vi "Logging Message Loop.vi"(8 "error in (no error)":T1 caption="entrée d'erreur (pas d'erreur)", 10 "File d'attente de données":refnum<queue>, 11 "Files d'attente de messages":T2) -> (0 "error out":T1 caption="sortie d'erreur")   [LabVIEW 2020, in "Logging.lvlib"]
doc: "Sous-VI de la boucle de messages qui gère les messages concernant l'enregistrement des données dans un fichier."
uses:
  Logging.lvlib
  support/Message Queue/All Message Queues.ctl
  support/Message Queue/Message Cluster.ctl
  Logging Configuration.ctl
  Logging State.ctl
  support/Message Queue/Enqueue Message (Single).vi
  <vilib>/Utility/error.llb/Error Cluster From Error Code.vi
  <vilib>/ErrorRing/Error Ring.xnode
  support/Message Queue/Message Queue.lvlib
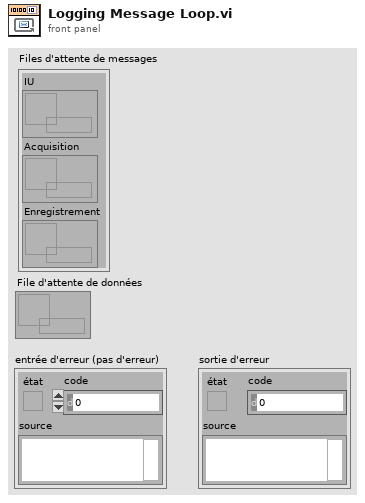
[diagram p1: front panel]
types:
  T1 = cluster{"état":bool, "code":i32, "source":string}
  T2 = typedef "Message Queue.lvlib/All Message Queues.ctl" = cluster{"IU":refnum<queue>, "Acquisition":refnum<queue>, "Enregistrement":refnum<queue>}
  T3 = typedef "Logging.lvlib/Logging Configuration.ctl" = cluster{"Chemin de base du fichier journal":path, "Référence de fichier TDMS":refnum<k34>}
  T4 = typedef "Logging.lvlib/Logging State.ctl" = enum16{"Idle", "Logging"}
  T5 = enum16{"open", "open or create", "create or replace", "create", "open (read-only)"}
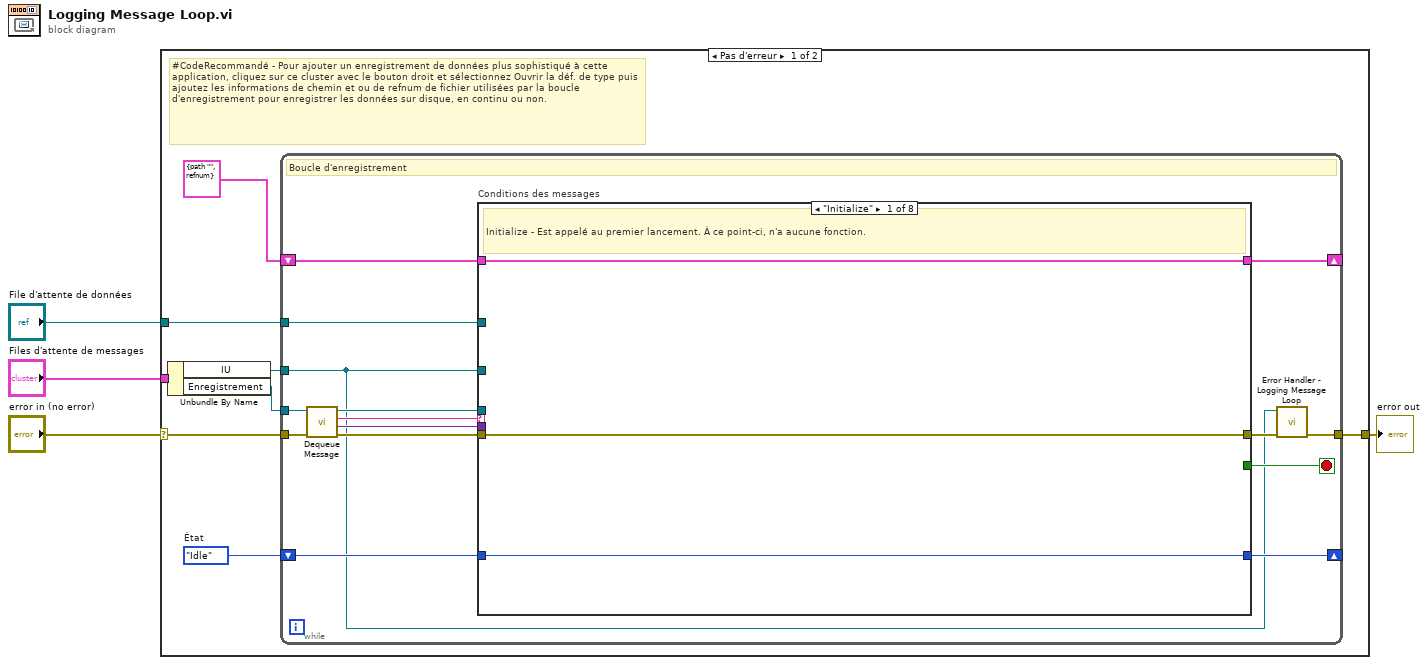
[diagram p0: block diagram]
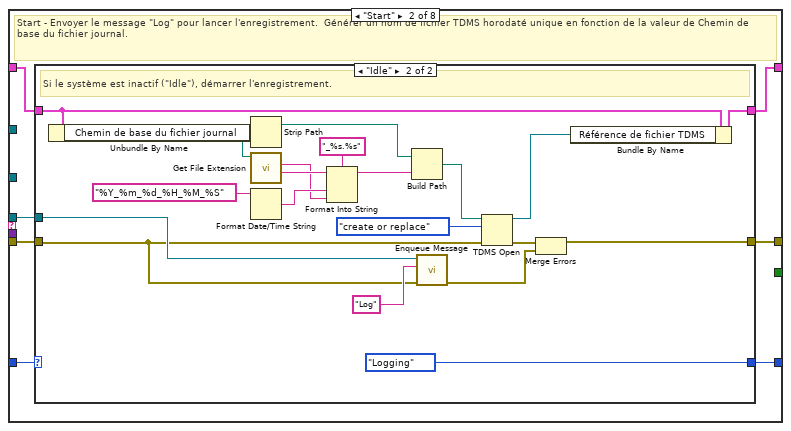
[diagram p2: hidden frame]
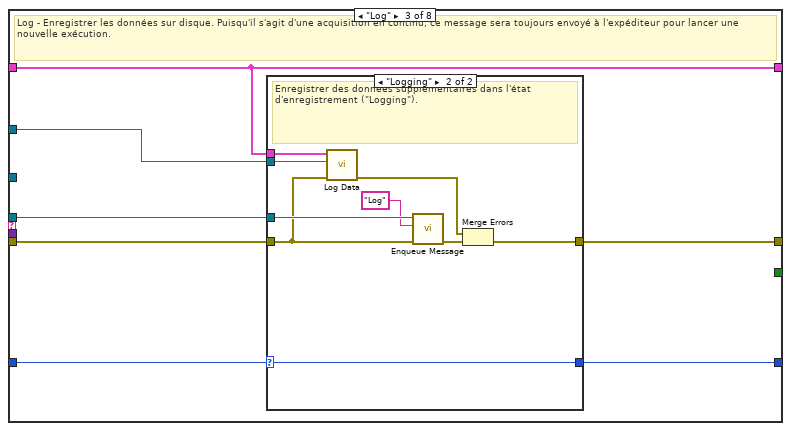
[diagram p4: hidden frame]
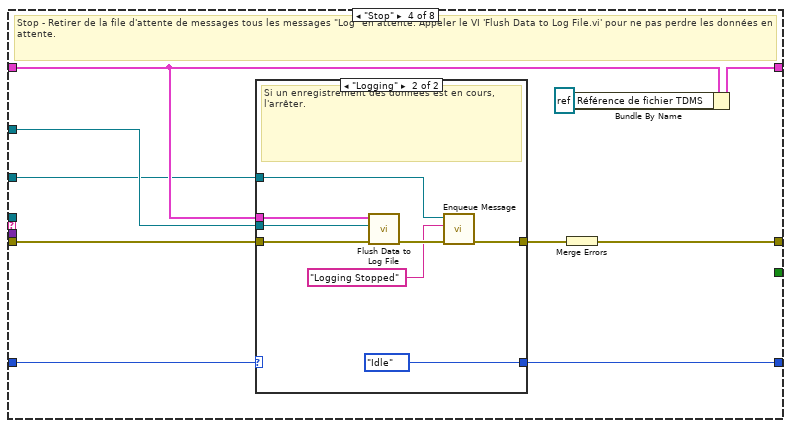
[diagram p6: hidden frame]
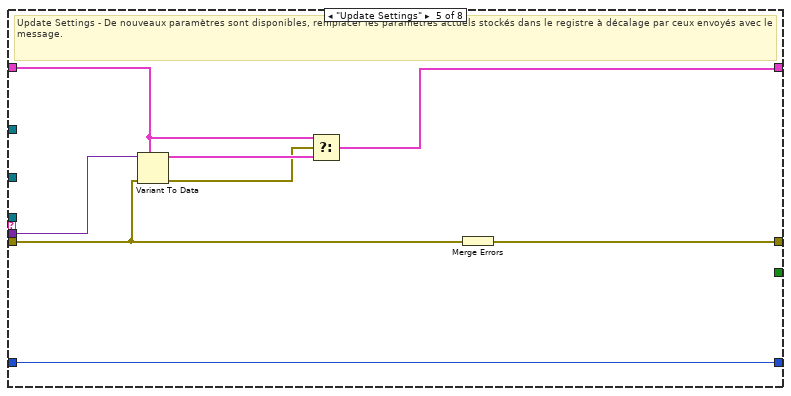
[diagram p8: hidden frame]
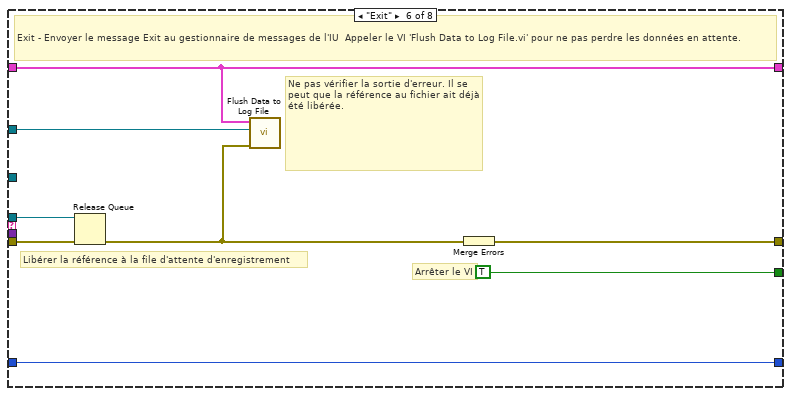
[diagram p9: hidden frame]
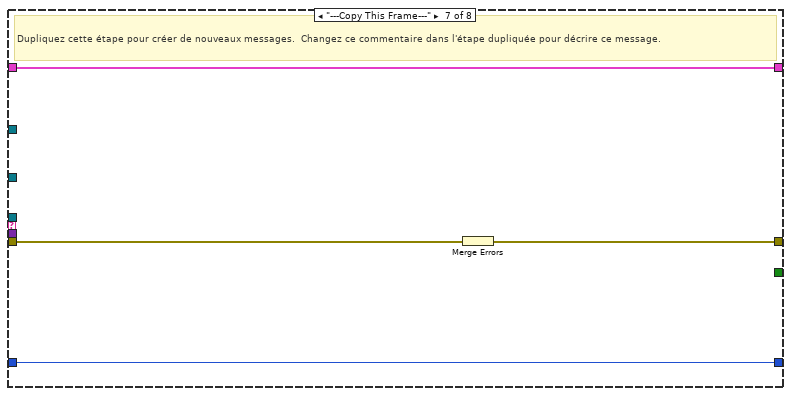
[diagram p10: hidden frame]
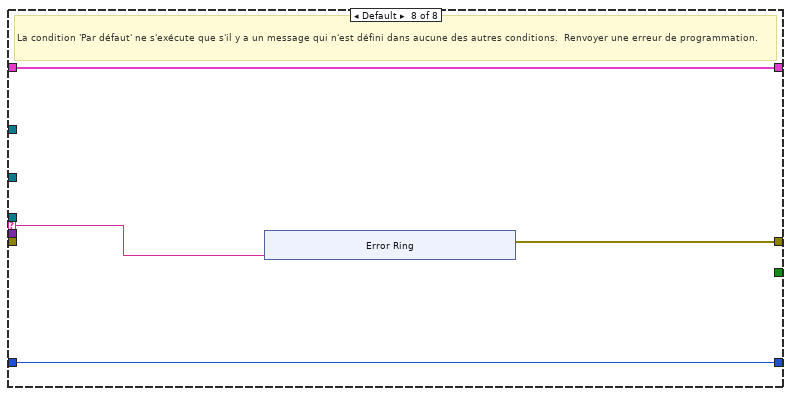
[diagram p11: hidden frame]
diagram:
  n1 = case shown="Pas d'erreur" "error in (no error)" {
    selector: "error in (no error)" -> [w8 w130]
    tunnel: "Files d'attente de messages" -> [w12 _]
    tunnel: [w10 w130] -> w3
    tunnel: "File d'attente de données" -> [w7 _]
    frame No Error {
      w5 = Logging_State."Idle"  # État
      # "#CodeRecommandé - Pour ajouter un enregistrement de données plus sophistiqué à cette application, cliquez sur ce cluster avec le bouton droit et sélectionnez Ouvrir la déf. de type puis ajoutez les informations de chemin et ou de refnum de fichier utilisées par la boucle d'enregistrement pour enregistrer les données sur disque, en continu ou non."
      n2 = Unbundle By Name(w12) -> ("IU"=w6:refnum<queue>, "Enregistrement"=w11:refnum<queue>)
      n3 = while {
        tunnel: w11 -> [w19]
        shift-right: [w26] -> _
        shift-left: T3 {"Chemin de base du fichier journal"=path "", "Référence de fichier TDMS"=refnum} ("Logging Configuration") -> [w27]
        tunnel: w6 -> [w13]
        tunnel: w7 -> [w18]
        shift-right: [w16] -> _
        shift-left: w5 -> [w17]
        tunnel: w8 -> [w24]
        tunnel: [w15] -> w10
        stop <- w25 stop-if-true
        # "Boucle d'enregistrement"
        n4 = call "Dequeue Message.vi"("error in (no error)"=w24, "File d'attente de messages"=w19) -> ("error out"=w23:T1, "Données de message"=w21:variant, "Message"=w22:string, "File d'attente de message dup."=w20:refnum<queue>)  [unwired: 6 in]
        n5 = case "Conditions des messages" shown="\"Initialize\"" w22 {
          selector: w22 -> [_ _ _ _ _ _ _ w119]
          tunnel: w20 -> [_ w36 w66 _ _ w111 _ _]
          tunnel: w23 -> [w29 w35 w64 w82 w100 w112 w118 _]
          tunnel: [w29 w37 w67 w88 w106 w113 w116 w120] -> w14
          tunnel: w27 -> [w30 w34 w63 w83 w104 w109 w117 w122]
          tunnel: [w30 w33 w63 w86 w101 w109 w117 w122] -> w26
          tunnel: [_ _ _ _ _ TRUE _ _] -> w25
          tunnel: w21 -> [_ _ _ _ w105 _ _ _]
          tunnel: w13 -> [_ _ _ w79 _ _ _ _]
          tunnel: w18 -> [_ _ w65 w84 _ w108 _ _]
          tunnel: w17 -> [w28 w32 w62 w81 w99 w107 w115 w121]
          tunnel: [w28 w31 w61 w80 w99 w107 w115 w121] -> w16
          frame "Initialize" {
            # "Initialize - Est appelé au premier lancement. À ce point-ci, n'a aucune fonction."
          }
          frame "Start" {
            # "Start - Envoyer le message \"Log\" pour lancer l'enregistrement.  Générer un nom de fichier TDMS horodaté unique en fonction de la valeur de Chemin de base du fichier journal."
            n6 = case shown="\"Idle\"" w32 {
              selector: w32 -> [w39 _]
              tunnel: [w38 w42] -> w37
              tunnel: w36 -> [_ w43]
              tunnel: w35 -> [w38 w41]
              tunnel: w34 -> [w40 w44]
              tunnel: [w40 w46] -> w33
              tunnel: [w39 Logging_State."Logging" ("State")] -> w31
              frame "Logging" {
                # "L'enregistrement des données est déjà en cours. Ignorer le message \"Start\"."
              }
              frame "Idle" {
                # "Si le système est inactif (\"Idle\"), démarrer l'enregistrement."
                n7 = Unbundle By Name(w44) -> ("Chemin de base du fichier journal"=w59:path)
                n8 = Strip Path(path=w59) -> (stripped path=w56:path)  [unwired: 1 out]
                n9 = call <vilib>:"Get File Extension.vi"("file"=w59) -> ("filename without extension"=w57:string, "lowercase file extension"=w53:string)  [unwired: 6 in, 3 out]
                n10 = Format Date/Time String(time format string (%c)="%Y_%m_%d_%H_%M_%S") -> (date/time string=w54:string)  [unwired: 2 in]
                n11 = Format Into String(format string="_%s.%s", initial string=w57, w54, w53) -> (resulting string=w52:string)  [unwired: 1 in, 1 out]
                n12 = Build Path(base path=w56, name or relative path=w52) -> (appended path=w51:path)
                n13 = call-poly "Enqueue Message.vi"("error in (no error)"=w41, "Message"="Log", "File d'attente de messages"=w43) -> ("error out"=w49:T1)  [unwired: 7 in, 1 out]
                n14 = TDMS Open(8:w41, 10:T5."create or replace" ("operation (0:open)"), 11:w51) -> (0:w50:errorcluster, 3:w47:refnum<k34>)  [unwired: 4 in]
                n15 = Merge Errors(w50, w49) -> (w42:errorcluster)
                n16 = Bundle By Name(cluster=w44, "Référence de fichier TDMS"=w47) -> (w46:T3)
              }
            }
          }
          frame "Log" {
            # "Log - Enregistrer les données sur disque. Puisqu'il s'agit d'une acquisition en continu, ce message sera toujours envoyé à l'expéditeur pour lancer une nouvelle exécution."
            n17 = case shown="\"Logging\"" w62 {
              selector: w62 -> [w69 w71]
              tunnel: [w68 w78] -> w67
              tunnel: w66 -> [_ w76]
              tunnel: w65 -> [_ w75]
              tunnel: w64 -> [w68 w70]
              tunnel: w63 -> [_ w72]
              tunnel: [w69 w71] -> w61
              frame "Idle" {
                # "Ignorer les messages \"Log\" quand l'enregistrement est inactif."
              }
              frame "Logging" {
                # "Enregistrer des données supplémentaires dans l'état d'enregistrement (\"Logging\")."
                n18 = call "Log Data.vi"("error in (no error)"=w70, "File d'attente de données"=w75, "Configuration de l'enregistrement"=w72) -> ("error out"=w74:T1)  [unwired: 8 in]
                n19 = call-poly "Enqueue Message.vi"("error in (no error)"=w70, "Message"="Log", "File d'attente de messages"=w76) -> ("error out"=w77:T1)  [unwired: 7 in, 1 out]
                n20 = Merge Errors(w74, w77) -> (w78:errorcluster)
              }
            }
          }
          frame "Stop" {
            # "Stop - Retirer de la file d'attente de messages tous les messages \"Log\" en attente. Appeler le VI 'Flush Data to Log File.vi' pour ne pas perdre les données en attente."
            n21 = case shown="\"Logging\"" w81 {
              selector: w81 -> [w89 _]
              tunnel: [w90 w93] -> w87
              tunnel: w84 -> [_ w97]
              tunnel: w83 -> [_ w96]
              tunnel: w82 -> [w90 w95]
              tunnel: [w89 Logging_State."Idle" ("State")] -> w80
              tunnel: w79 -> [_ w92]
              frame "Idle" {
                # "Le système est déjà inactif. Ignorer le message \"Stop\"."
              }
              frame "Logging" {
                # "Si un enregistrement des données est en cours, l'arrêter."
                n22 = call "Flush Data to Log File.vi"("error in (no error)"=w95, "File d'attente de données"=w97, "Configuration de l'enregistrement"=w96) -> ("error out"=w98:T1)  [unwired: 8 in]
                n23 = call-poly "Enqueue Message.vi"("error in (no error)"=w98, "Message"="Logging Stopped", "File d'attente de messages"=w92) -> ("error out"=w93:T1)  [unwired: 7 in, 1 out]
              }
            }
            n24 = Merge Errors(w87) -> (w88:errorcluster)
            n25 = Bundle By Name(cluster=w83, "Référence de fichier TDMS"=refnum<k34> refnum ("TDMS File Reference")) -> (w86:T3)
          }
          frame "Update Settings" {
            # "Update Settings - De nouveaux paramètres sont disponibles, remplacer les paramètres actuels stockés dans le registre à décalage par ceux envoyés avec le message."
            n26 = Variant To Data(error in=w100, type=w104, Variant=w105) -> (data=w103:T3, error out=w102:errorcluster)
            n27 = Select(t=w104, s=w102, f=w103) -> (s? t:f=w101:T3)
            n28 = Merge Errors(w100) -> (w106:errorcluster)
          }
          frame "Exit" {
            # "Ne pas vérifier la sortie d'erreur. Il se peut que la référence au fichier ait déjà été libérée."
            # "Libérer la référence à la file d'attente d'enregistrement"
            # "Arrêter le VI"
            # "Exit - Envoyer le message Exit au gestionnaire de messages de l'IU  Appeler le VI 'Flush Data to Log File.vi' pour ne pas perdre les données en attente."
            n29 = Release Queue(queue=w111, error in (no error)=w112) -> (error out=w110:errorcluster)  [unwired: 1 in, 2 out]
            n30 = call "Flush Data to Log File.vi"("error in (no error)"=w110, "File d'attente de données"=w108, "Configuration de l'enregistrement"=w109) -> ()  [unwired: 8 in, 1 out]
            n31 = Merge Errors(w110) -> (w113:errorcluster)
          }
          frame "---Copy This Frame---" {
            # "Dupliquez cette étape pour créer de nouveaux messages.  Changez ce commentaire dans l'étape dupliquée pour décrire ce message."
            n32 = Merge Errors(w118) -> (w116:errorcluster)
          }
          frame Default {
            # "La condition 'Par défaut' ne s'exécute que s'il y a un message qui n'est défini dans aucune des autres conditions.  Renvoyer une erreur de programmation."
            n33 = xnode ("Error Ring")("paramètre 0"=w119) -> ("sortie d'erreur"=w120:errorcluster)
          }
        }
        n34 = call "Error Handler - Logging Message Loop.vi"("error in (no error)"=w14, "File d'attente de messages"=w13) -> ("erreur en entrée dup."=w15:T1)  [unwired: 8 in, 1 out]
      }
    }
    frame Error {
    }
  }
  "error out" <- w3
